vi "fgv_sensor-data.vi"() -> ()   [LabVIEW 2021]
uses:
  ctrl/init-r-update.ctl
panel:
  in  "cmd":T1
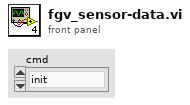
[diagram p1: front panel]
types:
  T1 = typedef "init-r-update.ctl" = enum16{"init", "read", "update"}
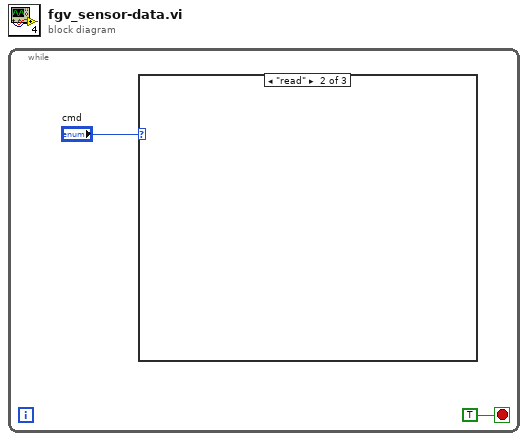
[diagram p0: block diagram]
diagram:
  n1 = while {
    stop <- TRUE stop-if-true
    n2 = case shown="\"read\"" "cmd" {
      frame "init", Default {
      }
      frame "read" {
      }
      frame "update" {
      }
    }
  }
